vi "消息推送.vi"(8 "error in (no error)":errorcluster caption="错误输入（无错误）", 9 "数据内容":string="1、建议排查管路是否异常\n2、供电情况是否正常", 10 "参数":string="故障告警", 11 "站点":string="测试点") -> (0 "error out":errorcluster caption="错误输出")   [LabVIEW 2016, in "wxpusher.lvlib"]
uses:
  wxpusher.lvlib
  <vilib>/Utility/error.llb/DialogType.ctl
panel:
  out "GBK":string
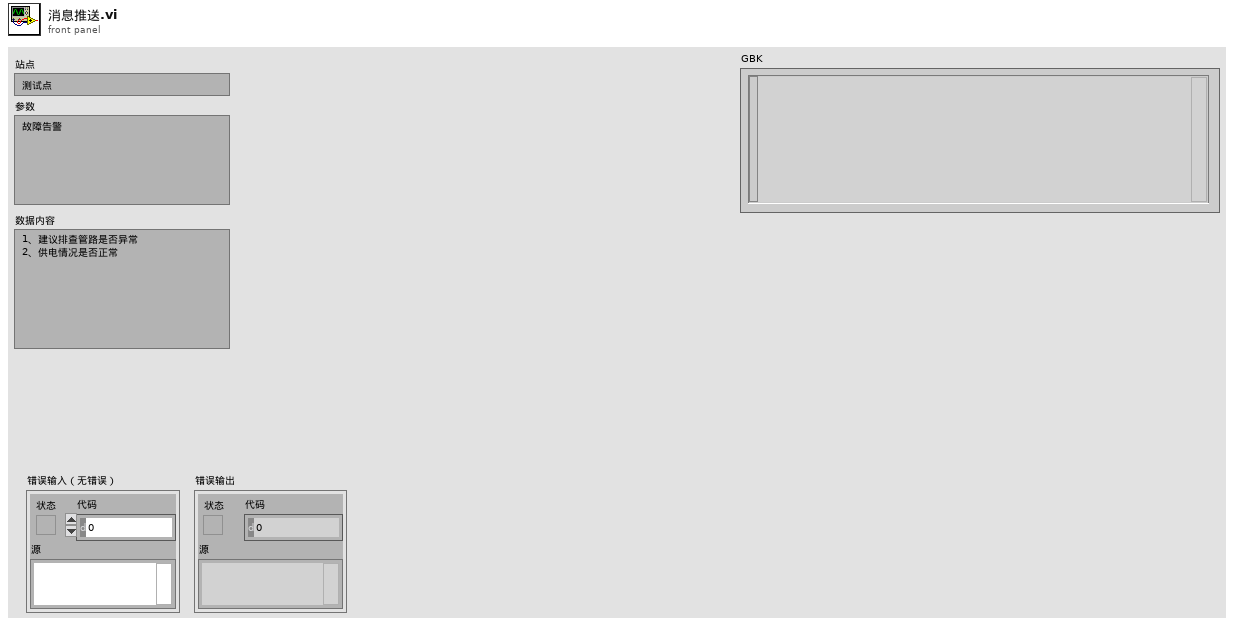
[diagram p1: front panel]
types:
  T1 = typedef "DialogType.ctl" = u16
  T2 = cluster{"action":string, "data":cluster{"appKey":string, "appName":string, "source":string, "time":u64, "uid":string, "userHeadImg":string, "userName":string, "extra":string}}[]
  T3 = enum16{"open", "replace", "create", "open or create", "replace or create", "replace or create with confirmation"}
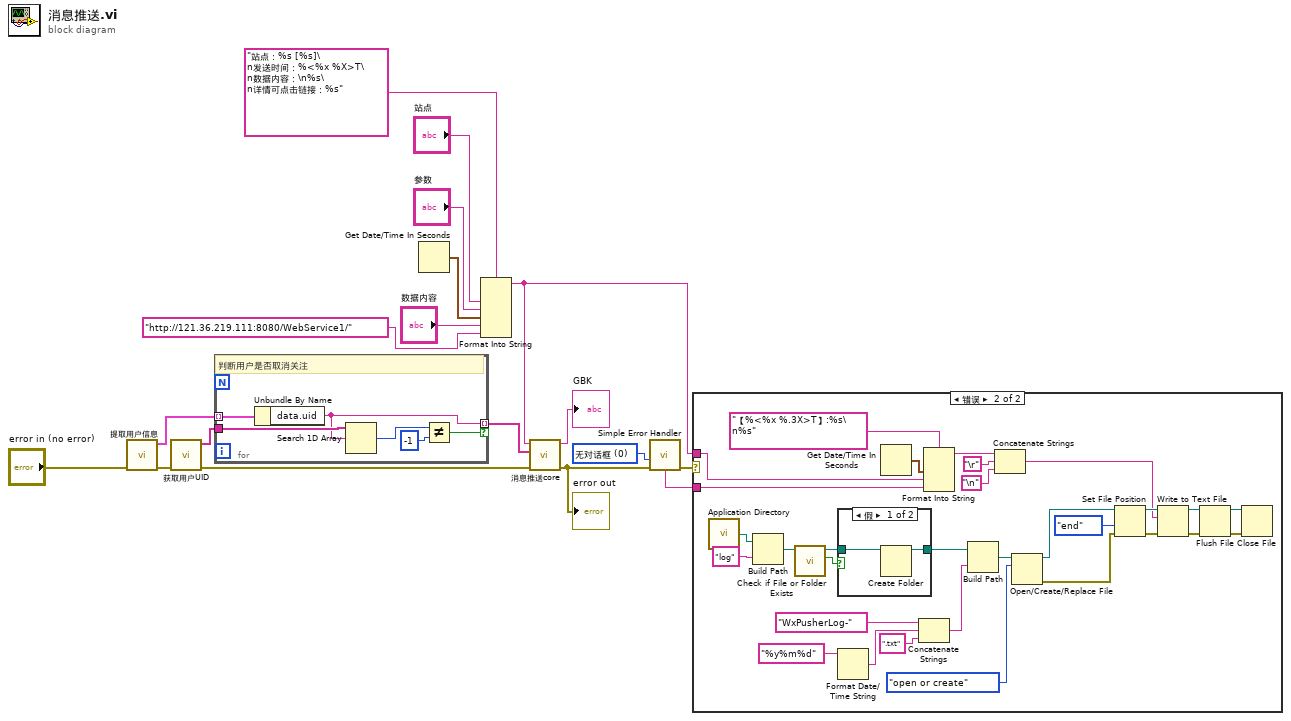
[diagram p0: block diagram]
diagram:
  w5 = T1 0 items=["无对话框", "确定信息", "继续或停止信息", "确定信息＋警告", "继续/停止+警告"] ("type of dialog (OK msg:1)")
  n1 = call "提取用户信息.vi"("error in (no error)"="error in (no error)") -> ("error out"=w13:errorcluster, "用户信息"=w18:T2)  [unwired: 9 in]
  n2 = call "获取用户UID.vi"("error in (no error)"=w13) -> ("error out"=w11:errorcluster, "uid"=w12:string[])  [unwired: 9 in]
  n3 = for {
    tunnel: w18 -> [w24] mode=indexing
    tunnel: [w22] -> w17 mode=indexing if=w19
    tunnel: w12 -> [w23]
    # "判断用户是否取消关注"
    n4 = Unbundle By Name(w24) -> ("data.uid"=w22:string)
    n5 = Search 1D Array(1D array=w23, element=w22) -> (index of element=w21:i32)  [unwired: 1 in]
    n6 = Not Equal?(x=w21, y=-1) -> (x != y?=w19:bool)
  }
  n7 = Get Date/Time In Seconds() -> (seconds since 1Jan1904=w15:timestamp)
  n8 = Format Into String(format string="站点：%s [%s]\n发送时间：%<%x %X>T\n数据内容：\n%s\n详情可点击链接：%s" ("格式字符串"), "站点", "参数", w15, "数据内容", "http://121.36.219.111:8080/WebService1/" ("输入 5")) -> (resulting string=w2:string)  [unwired: 2 in, 1 out]
  n9 = call "消息推送core.vi"("error in (no error)"=w11, "数组"=w17, "content"=w2) -> ("error out"=w6:errorcluster, "GBK"=→"GBK":string)  [unwired: 7 in]
  "error out" <- w6
  n10 = call <vilib>:"Simple Error Handler.vi"("type of dialog (OK msg:1)"=w5, "error in (no error)"=w6) -> ("error out"=w3:errorcluster, "message"=w4:string)  [unwired: 3 in, 3 out]
  n11 = case shown="错误" w3 {
    tunnel: w4 -> [_ w26]
    tunnel: w2 -> [_ w25]
    frame No Error {
    }
    frame Error {
      n12 = call <vilib>:"Application Directory.vi"() -> ("Application Directory"=w33:path)
      n13 = Build Path(base path=w33, name or relative path="log" ("名称或相对路径")) -> (appended path=w31:path)
      n14 = call <vilib>:"Check if File or Folder Exists.vi"("path"=w31) -> ("file or folder exists?"=w46:bool, "dup path"=w45:path)  [unwired: 8 in, 1 out]
      n15 = case shown="假" w46 {
        tunnel: w45 -> [w56 w57]
        tunnel: [w55 w57] -> w44
        frame False {
          n16 = Create Folder(path (use dialog)=w56) -> (created path=w55:path)  [unwired: 2 in, 2 out]
        }
        frame True {
        }
      }
      n17 = Format Date/Time String(time format string (%c)="%y%m%d" ("时间格式字符串(%c)")) -> (date/time string=w42:string)  [unwired: 2 in]
      n18 = Get Date/Time In Seconds() -> (seconds since 1Jan1904=w53:timestamp)
      n19 = Concatenate Strings("WxPusherLog-" ("字符串"), w42, ".txt" ("字符串")) -> (w41:string)
      n20 = Format Into String(format string="【%<%x %.3X>T】:%s\n%s" ("格式字符串"), w53, w25, w26) -> (resulting string=w52:string)  [unwired: 2 in, 1 out]
      n21 = Build Path(base path=w44, name or relative path=w41) -> (appended path=w40:path)
      n22 = Concatenate Strings(w52, "\r", "\n") -> (w29:string)
      n23 = Open/Create/Replace File(file path (use dialog)=w40, operation (0:open)=T3."open or create" ("操作(0:open)")) -> (refnum out=w48:refnum<file>, error out=w50:errorcluster)  [unwired: 4 in, 1 out]
      n24 = Set File Position(refnum=w48, from (0:start)=enum16{"start", "end", "current"}."end" ("自（0:起始）"), error in=w50) -> (refnum out=w49:refnum<file>, error out=w51:errorcluster)  [unwired: 1 in]
      n25 = Write to Text File(file (use dialog)=w49, text=w29, error in=w51) -> (refnum out=w36:refnum<file>, error out=w35:errorcluster)  [unwired: 1 in, 1 out]
      n26 = Flush File(refnum=w36, error in=w35) -> (refnum out=w38:refnum<file>, error out=w37:errorcluster)
      n27 = Close File(refnum=w38, error in=w37) -> ()  [unwired: 2 out]
    }
  }
